vi "ECC write.vi"(9 "Address":dbl, 10 "Parameter code":dbl, 11 "Value":dbl=1000.0) -> (2 "Data array":dbl[](array[numeric]))   [LabVIEW 2010, in "Yudian AI508.lvlib"]
uses:
  <instrlib>/Yudian AI508/Yudian AI508.lvlib
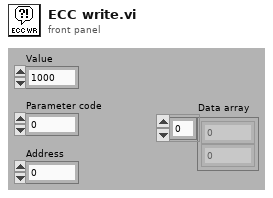
[diagram p1: front panel]
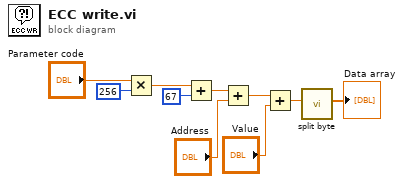
[diagram p0: block diagram]
diagram:
  n1 = Multiply(x="Parameter code", y=256) -> (x*y=w8:dbl)
  n2 = Add(x=w8, y=67) -> (x+y=w6:dbl)
  n3 = Add(x=w6, y="Address") -> (x+y=w3:dbl)
  n4 = Add(x=w3, y="Value") -> (x+y=w1:dbl)
  n5 = call <instrlib>:"split byte.vi"("Value"=w1) -> ("Array"=→"Data array":dbl[])  [unwired: 10 in]
